vi "CT_VFModifyPuffTrig.vi"(1 "Reference Index":i32=1, 2 "Extra Delay (us)":dbl, 3 "Delay Index":i32, 4 "Very Fast Timing In":dbl[](array[slide])=[1100.0, 3200.0, 3254.0, 3290.0, 3100.0, 3080.0, 0.0, 3100.0] min=0.0 max=4000.0 step=2.0 scale=0.0..4000.0 scale format="%#_3f") -> (0 "Very Fast Timing Out":dbl[](array[slide])=[1100.0, 3200.0, 3254.0, 3290.0, 3100.0, 3080.0, 0.0, 3100.0] min=0.0 max=4000.0 step=2.0 scale=0.0..4000.0 scale format="%#_3f")   [LabVIEW 2016]
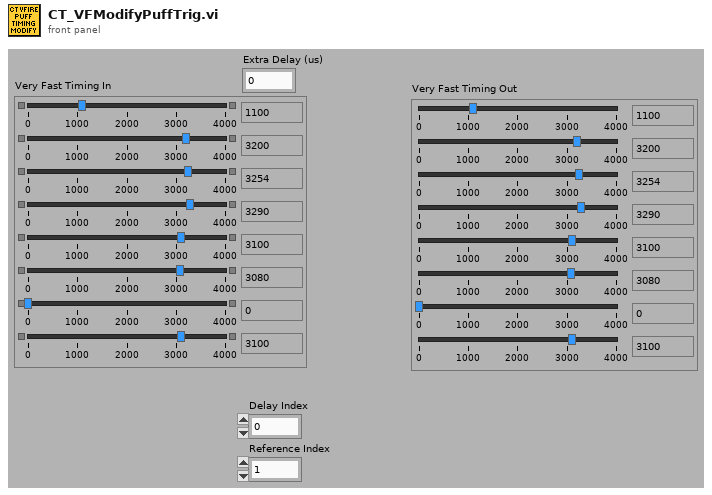
[diagram p1: front panel]
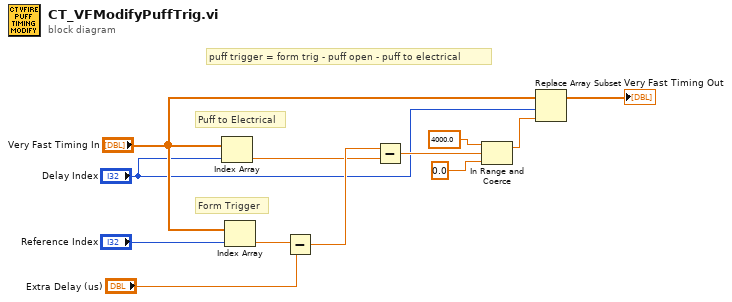
[diagram p0: block diagram]
diagram:
  # "puff trigger = form trig - puff open - puff to electrical"
  # "Form Trigger"
  # "Puff to Electrical"
  n1 = Index Array(array="Very Fast Timing In", index="Delay Index") -> (element=w8:dbl)
  n2 = Index Array(array="Very Fast Timing In", index="Reference Index") -> (element=w11:dbl)
  n3 = Subtract(x=w11, y="Extra Delay (us)") -> (x-y=w9:dbl)
  n4 = Subtract(x=w9, y=w8) -> (x-y=w5:dbl)
  n5 = In Range and Coerce(upper limit=4000.0, x=w5, lower limit=0.0) -> (coerced(x)=w4:dbl)  [unwired: 1 out]
  n6 = Replace Array Subset(array="Very Fast Timing In", new element=w4, index="Delay Index") -> (→"Very Fast Timing Out":dbl[])
